vi "SIM921_Open_Queue.vi"(8 "error in (no error)":errorcluster) -> (0 "error out":errorcluster, 2 "queue out":refnum<queue>)   [LabVIEW 2019]
uses:
  SIM921/SIM921_control_cluster.ctl
  Global/Global Variables/Queues_global.vi
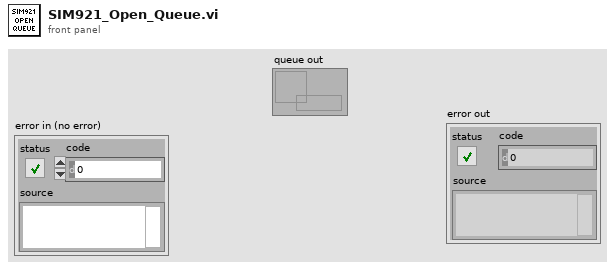
[diagram p1: front panel]
types:
  T1 = typedef "SIM921_control_cluster.ctl" = cluster{"Update":bool}
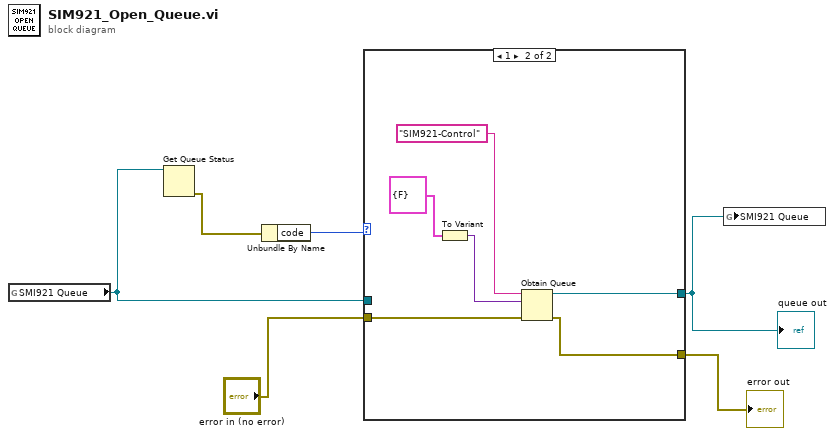
[diagram p0: block diagram]
diagram:
  n1 = global read "Queues_global.vi" "SMI921 Queue"() -> (w6:refnum<queue>)
  n2 = Get Queue Status(queue=w6) -> (error out=w5:errorcluster)  [unwired: 2 in, 7 out]
  n3 = Unbundle By Name(w5) -> ("code"=w4:i32)
  n4 = case shown="1" w4 {
    tunnel: w6 -> [w8 _]
    tunnel: [w8 w11] -> w3
    tunnel: "error in (no error)" -> [w7 w10]
    tunnel: [w7 w9] -> w1
    frame 0, Default {
    }
    frame 1 {
      n5 = To Variant(anything=T1 {"Update"=FALSE} ("SIM921-Control")) -> (Variant=w13:variant)
      n6 = Obtain Queue(name (unnamed)="SIM921-Control", element data type=w13, error in (no error)=w10) -> (queue out=w11:refnum<queue>, error out=w9:errorcluster)  [unwired: 2 in, 1 out]
    }
  }
  "queue out" <- w3
  "error out" <- w1
  n7 = global write "Queues_global.vi" "SMI921 Queue"(w3) -> ()
